vi "Detect Gait Events.vi"(5 "GPD Parameters":T5, 6 "Event Data in":T8, 7 "Gyro Data":T2) -> (1 "GPD Parameters":T5, 2 "Event Data out":T8, 3 "Event Data for Log and Plot":T1)   [LabVIEW 2019]
uses:
  Controls/Event Data.ctl
  Controls/Side Event Data.ctl
  Controls/GPD Parameters.ctl
  Controls/GPD Parameter Names.ctl
  Controls/GPD Side Parameters.ctl
  Controls/Gyro Data.ctl
  Controls/Gyro Side Data.ctl
  Controls/Gyro Negation.ctl
  Controls/Event Data for Plot and Log.ctl
panel:
  out "Gyro Z":cluster{"Left Gyro Z":dbl, "Right Gyro Z":dbl}
  out "Gyro Data":T2
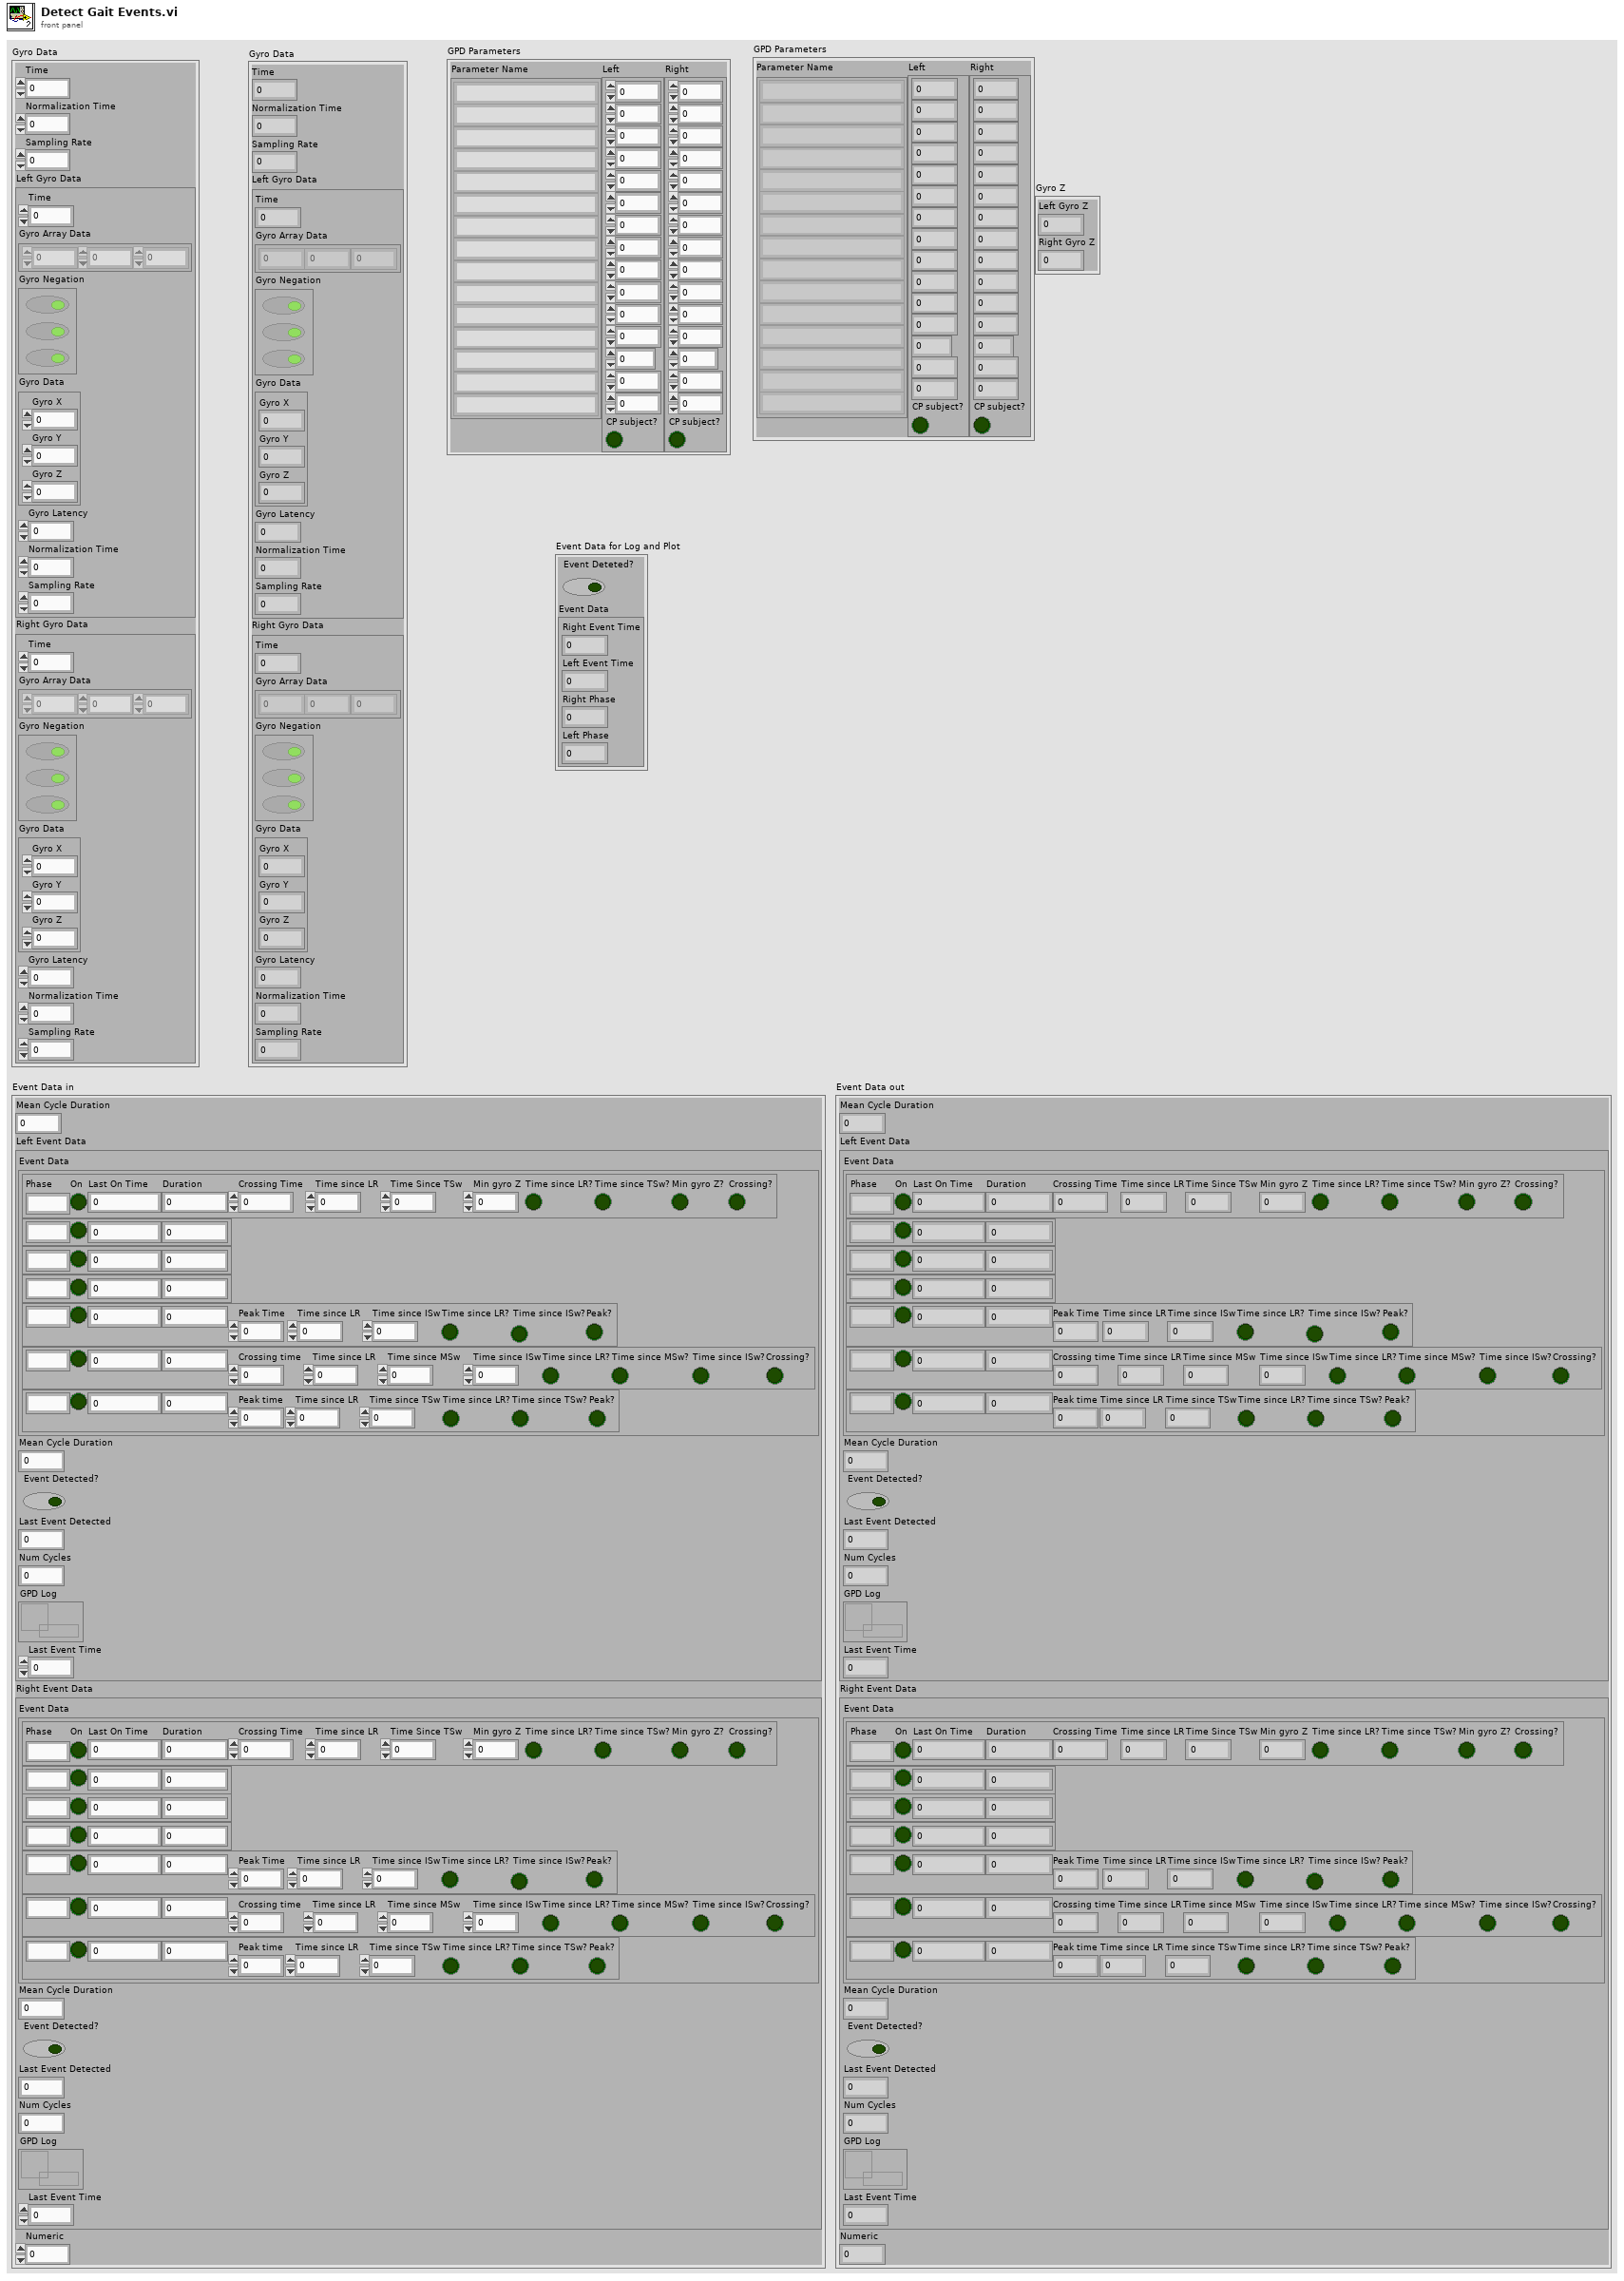
[diagram p1: front panel]
types:
  T1 = typedef "Event Data for Plot and Log.ctl" = cluster{"Event Deteted?":bool, "Event Data":cluster{"Right Event Time":dbl, "Left Event Time":dbl, "Right Phase":i32, "Left Phase":i32}}
  T2 = typedef "Gyro Data.ctl" = cluster{"Time":dbl, "Normalization Time":dbl, "Sampling Rate":dbl, "Left Gyro Data":T3, "Right Gyro Data":T3}
  T3 = typedef "Gyro Side Data.ctl" = cluster{"Time":dbl, "Gyro Array Data":dbl[], "Gyro Negation":T4, "Gyro Data":cluster{"Gyro X":dbl, "Gyro Y":dbl, "Gyro Z":dbl}, "Gyro Latency":dbl, "Normalization Time":dbl, "Sampling Rate":dbl}
  T4 = typedef "Gyro Negation.ctl" = bool[]
  T5 = typedef "GPD Parameters.ctl" = cluster{"Parameter Name":T6, "Left":T7, "Right":T7}
  T6 = typedef "GPD Parameter Names.ctl" = string[]
  T7 = typedef "GPD Side Parameters.ctl" = cluster{"% Cycle Delay":dbl, "Min % Cycle LR to ISw ":dbl, "Min % Cycle LR to MSw":dbl, "Min % Cycle LR to TSw":dbl, "Max % Cycle ISw to MSw":dbl, "Min % Cycle TSw to LR":dbl, "Max % Cycle TSw to LR":dbl, "LR Min Gyro Z Threshold":dbl, "LR Min Gyro Z Width":dbl, "ISw Peak Threshold":dbl, "ISw Peak Width":dbl, "TSw Valley Threshold":dbl, "TSw Valley Width (ms)":dbl, "Max Cycle Time (s)":dbl, "Mean Computation Window":dbl, "CP subject?":bool}
  T8 = typedef "Event Data.ctl" = cluster{"Mean Cycle Duration":dbl, "Left Event Data":T9, "Right Event Data":T9, "Numeric":dbl}
  T9 = typedef "Side Event Data.ctl" = cluster{"Event Data":cluster{"LR":cluster{"Phase":string, "On":bool, "Last On Time":dbl, "Duration":dbl, "Crossing Time":dbl, "Time since LR":dbl, "Time Since TSw":dbl, "Min gyro Z":dbl, "Time since LR?":bool, "Time since TSw?":bool, "Min gyro Z?":bool, "Crossing?":bool}, "MSt":cluster{"Phase":string, "On":bool, "Last On Time":dbl, "Duration":dbl}, "TSt":cluster{"Phase":string, "On":bool, "Last On Time":dbl, "Duration":dbl}, "PSw":cluster{"Phase":string, "On":bool, "Last On Time":dbl, "Duration":dbl}, "ISw":cluster{"Phase":string, "On":bool, "Last On Time":dbl, "Duration":dbl, "Peak Time":dbl, "Time since LR":dbl, "Time since ISw":dbl, "Time since LR?":bool, "Time since ISw?":bool, "Peak?":bool}, "MSw":cluster{"Phase":string, "On":bool, "Last On Time":dbl, "Duration":dbl, "Crossing time":dbl, "Time since LR":dbl, "Time since MSw":dbl, "Time since ISw":dbl, "Time since LR?":bool, "Time since MSw?":bool, "Time since ISw?":bool, "Crossing?":bool}, "TSw":cluster{"Phase":string, "On":bool, "Last On Time":dbl, "Duration":dbl, "Peak time":dbl, "Time since LR":dbl, "Time since TSw":dbl, "Time since LR?":bool, "Time since TSw?":bool, "Peak?":bool}}, "Mean Cycle Duration":dbl, "Event Detected?":bool, "Last Event Detected":i32, "Num Cycles":dbl, "GPD Log":refnum<queue>, "Last Event Time":dbl}
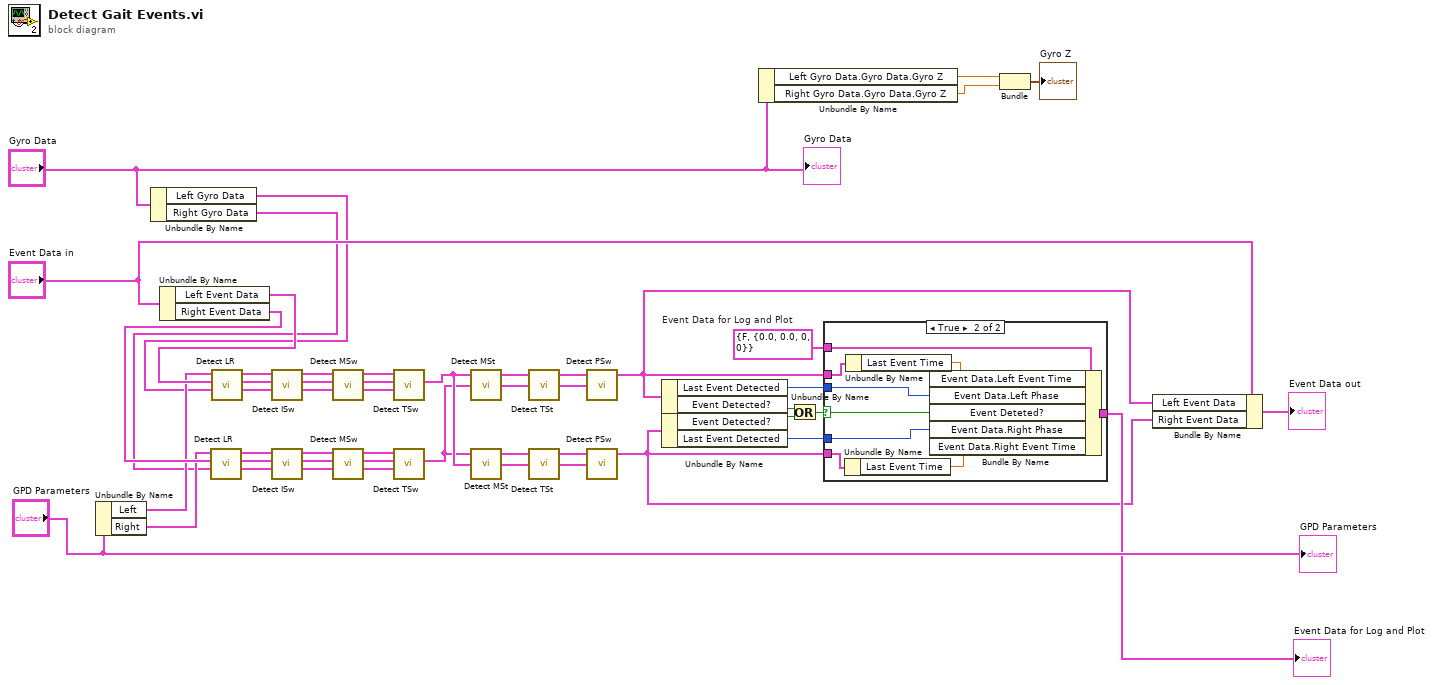
[diagram p0: block diagram]
diagram:
  w8 = T1 {"Event Deteted?"=FALSE, "Event Data"={"Right Event Time"=0.0, "Left Event Time"=0.0, "Right Phase"=0, "Left Phase"=0}}  # Event Data for Log and Plot
  n1 = Unbundle By Name("GPD Parameters") -> ("Left"=w45:T7, "Right"=w46:T7)
  n2 = Unbundle By Name("Gyro Data") -> ("Left Gyro Data"=w43:T3, "Right Gyro Data"=w42:T3)
  n3 = Unbundle By Name("Event Data in") -> ("Left Event Data"=w48:T9, "Right Event Data"=w47:T9)
  n4 = call "Detect LR.vi"("Side Gyro Data"=w42, "Side Event Data"=w47, "GPD Parameters"=w46) -> ("Side Gyro Data"=w39:T3, "Side Event Data"=w36:T9, "GPD Parameters"=w19:T7)  [unwired: 5 in, 1 out]
  n5 = call "Detect LR.vi"("Side Gyro Data"=w43, "Side Event Data"=w48, "GPD Parameters"=w45) -> ("Side Gyro Data"=w27:T3, "Side Event Data"=w24:T9, "GPD Parameters"=w14:T7)  [unwired: 5 in, 1 out]
  n6 = call "Detect ISw.vi"("Side Gyro Data"=w27, "Side Event Data"=w24, "GPD Parameters"=w14) -> ("Side Gyro Data"=w28:T3, "Side Event Data"=w25:T9, "GPD Parameters"=w15:T7)  [unwired: 5 in, 1 out]
  n7 = call "Detect ISw.vi"("Side Gyro Data"=w39, "Side Event Data"=w36, "GPD Parameters"=w19) -> ("Side Gyro Data"=w40:T3, "Side Event Data"=w37:T9, "GPD Parameters"=w20:T7)  [unwired: 5 in, 1 out]
  n8 = call "Detect MSw.vi"("Side Gyro Data"=w28, "Side Event Data"=w25, "GPD Parameters"=w15) -> ("Gyro Data Out"=w29:T3, "Side Event Data"=w26:T9, "GPD Parameters out"=w16:T7)  [unwired: 5 in, 1 out]
  n9 = call "Detect MSw.vi"("Side Gyro Data"=w40, "Side Event Data"=w37, "GPD Parameters"=w20) -> ("Gyro Data Out"=w41:T3, "Side Event Data"=w38:T9, "GPD Parameters out"=w21:T7)  [unwired: 5 in, 1 out]
  n10 = call "Detect TSw.vi"("Side Gyro Data"=w29, "Side Event Data"=w26, "GPD Parameters"=w16) -> ("Side Event Data"=w23:T9)  [unwired: 5 in, 3 out]
  n11 = call "Detect TSw.vi"("Side Gyro Data"=w41, "Side Event Data"=w38, "GPD Parameters"=w21) -> ("Side Event Data"=w22:T9)  [unwired: 5 in, 3 out]
  n12 = call "Detect MSt.vi"("Contralateral Event Data"=w22, "Ipsilateral Event Data"=w23) -> ("Contralateral Event Data"=w30:T9, "Ipsilateral Event Data"=w17:T9)  [unwired: 2 in]
  n13 = call "Detect MSt.vi"("Contralateral Event Data"=w23, "Ipsilateral Event Data"=w22) -> ("Contralateral Event Data"=w34:T9, "Ipsilateral Event Data"=w32:T9)  [unwired: 2 in]
  n14 = call "Detect TSt.vi"("Contralateral Event Data"=w30, "Ipsilateral Event Data"=w17) -> ("Contralateral Event Data"=w31:T9, "Ipsilateral Event Data"=w18:T9)  [unwired: 2 in]
  n15 = call "Detect TSt.vi"("Contralateral Event Data"=w34, "Ipsilateral Event Data"=w32) -> ("Contralateral Event Data"=w35:T9, "Ipsilateral Event Data"=w33:T9)  [unwired: 2 in]
  n16 = call "Detect PSw.vi"("Contralateral Event Data"=w31, "Ipsilateral Event Data"=w18) -> ("Ipsilateral Event Data"=w6:T9)  [unwired: 2 in, 1 out]
  n17 = call "Detect PSw.vi"("Contralateral Event Data"=w35, "Ipsilateral Event Data"=w33) -> ("Ipsilateral Event Data"=w5:T9)  [unwired: 2 in, 1 out]
  n18 = Unbundle By Name(w6) -> ("Last Event Detected"=w10:i32, "Event Detected?"=w13:bool)
  n19 = Unbundle By Name(w5) -> ("Event Detected?"=w12:bool, "Last Event Detected"=w9:i32)
  n20 = Unbundle By Name("Gyro Data") -> ("Left Gyro Data.Gyro Data.Gyro Z"=w3:dbl, "Right Gyro Data.Gyro Data.Gyro Z"=w2:dbl)
  n21 = Or(x=w13, y=w12) -> (x .or. y?=w11:bool)
  n22 = case shown="True" w11 {
    selector: w11 -> [_ w54]
    tunnel: w6 -> [_ w60]
    tunnel: w5 -> [_ w59]
    tunnel: w10 -> [_ w56]
    tunnel: w9 -> [_ w55]
    tunnel: [w51 w53] -> w7
    tunnel: w8 -> [w51 w52]
    frame False {
    }
    frame True {
      n23 = Unbundle By Name(w59) -> ("Last Event Time"=w57:dbl)
      n24 = Unbundle By Name(w60) -> ("Last Event Time"=w58:dbl)
      n25 = Bundle By Name(cluster=w52, "Event Data.Left Event Time"=w58, "Event Data.Left Phase"=w56, "Event Deteted?"=w54, "Event Data.Right Phase"=w55, "Event Data.Right Event Time"=w57) -> (w53:T1)
    }
  }
  "Event Data for Log and Plot" <- w7
  n26 = Bundle("Gyro Z"=w3, "Gyro Z"=w2) -> (→"Gyro Z":cluster{"Gyro Z":dbl, "Gyro Z":dbl})  [unwired: 1 in]
  n27 = Bundle By Name(cluster="Event Data in", "Left Event Data"=w6, "Right Event Data"=w5) -> (→"Event Data out":T8)
  "GPD Parameters" <- "GPD Parameters"
  "Gyro Data" <- "Gyro Data"
